vi "Filter From Source(Queue).vi"() -> ()   [LabVIEW 2017, in "CSM Global Log Filter Example.lvlib"]
uses:
  user.lib/_NEVSTOP/Communicable State Machine(CSM)/_Support/Typedef/_CSM_GlobalLog Filter Rules - v1.0.ctl
  user.lib/_NEVSTOP/Communicable State Machine(CSM)/_Support/Typedef/_CSM_GlobalLog_MSG_TYPE.ctl
  user.lib/_NEVSTOP/Communicable State Machine(CSM)/_Support/Typedef/_CSM_GlobalLog_STATE_TYPE.ctl
  user.lib/_NEVSTOP/Communicable State Machine(CSM)/Utility/_support/Periodic String Filter Level.ctl
  user.lib/_NEVSTOP/Communicable State Machine(CSM)/Utility/Periodic String Filter Setting.ctl
  user.lib/_NEVSTOP/Communicable State Machine(CSM)/_Support/GlobalEvent/GEvt-Set Source Filter Rules - v1.0.vi
  CSM Global Log Filter Example.lvlib
  user.lib/_NEVSTOP/Communicable State Machine(CSM)/Communicable State Machine.lvlib
  1. Create a reuse Module/1. Create a reuse Module.lvlib
  user.lib/_NEVSTOP/Communicable State Machine(CSM)/_Shared/CSM Shared.lvlib
panel:
  out "LogInQ":i32
  out "State History":string
  out "log handling Speed(#/s)":dbl
  out "LogInQ changing Speed(#/s)":dbl
  out "Level":T1
  in  "Stop":bool
  in  "Rules-v1":T2={"Global"={"CSM"=["Module2"], "LogType"=[], "State"=[], "StateType"=[]}, "CSM"={"LogType"=[{"CSM"="Module1", "LogType"=enum."State Change"}], "State"=[{"CSM"="Module3", "State"=""}], "StateType"=[]}}
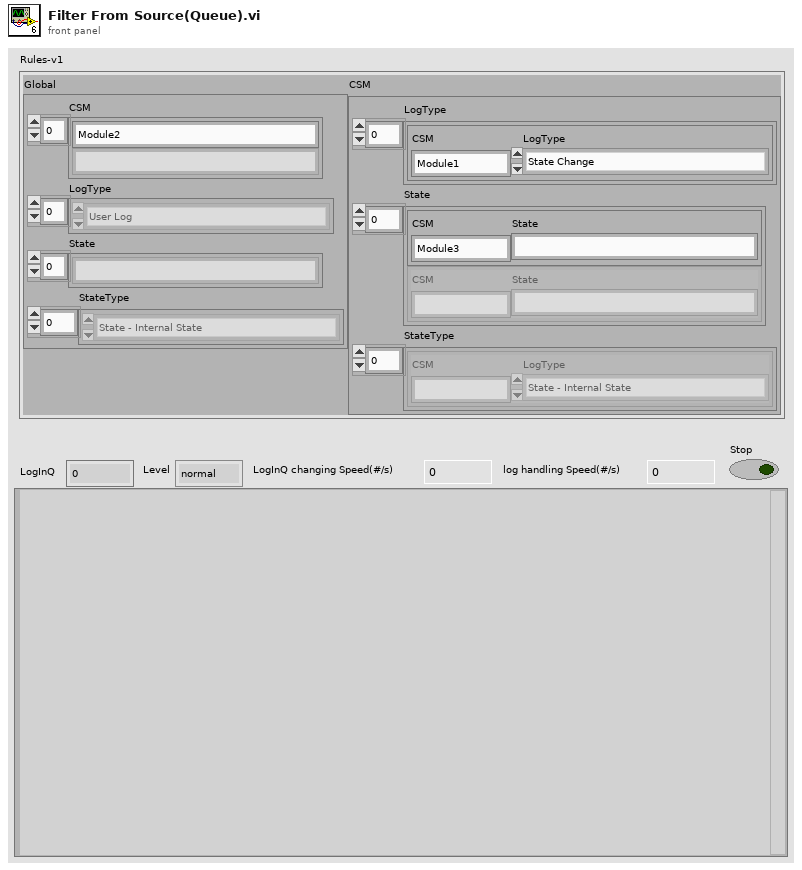
[diagram p1: front panel]
types:
  T1 = typedef "Communicable State Machine.lvlib/Periodic String Filter Level.ctl" = enum16{"normal", "L1", "L2", "L3", "L4"}
  T2 = typedef "Communicable State Machine.lvlib/_CSM_GlobalLog Filter Rules - v1.0.ctl" = cluster{"Global":cluster{"CSM":string[], "LogType":T3[], "State":string[], "StateType":T4[]}, "CSM":cluster{"LogType":cluster{"CSM":string, "LogType":T3}[], "State":cluster{"CSM":string, "State":string}[], "StateType":cluster{"CSM":string, "LogType":T4}[]}}
  T3 = typedef "Communicable State Machine.lvlib/_CSM_GlobalLog_MSG_TYPE.ctl" = enum16{"User Log", "State Change", "Status", "Interrupt", "Register", "Unregister", "Error Log", "Module Created", "Module Destroyed"}
  T4 = typedef "Communicable State Machine.lvlib/_CSM_GlobalLog_STATE_TYPE.ctl" = enum16{"State - Internal State", "State - External Message", "State - Response", "State - Complete"}
  T5 = typedef "Communicable State Machine.lvlib/Periodic String Filter Setting.ctl" = cluster{"threashold(#/s)":dbl, "Check Peroid(s)":dbl}
  T6 = typedef "Communicable State Machine.lvlib/_CSM_GlobalLog_MSG.ctl" = cluster{"Name (\"\" to Use UUID)":string, "Current State":string, "Arguments":string, "Source Message":T7, "Source Module":string, "Complete(T)/Start(F)":bool, "LogType":T3, "Time Stamp":timestamp}
  T7 = typedef "Communicable State Machine.lvlib/_CSM_Response Source Message.ctl" = cluster{"‘State":string, "’Arguments":string, "’Error":errorcluster}
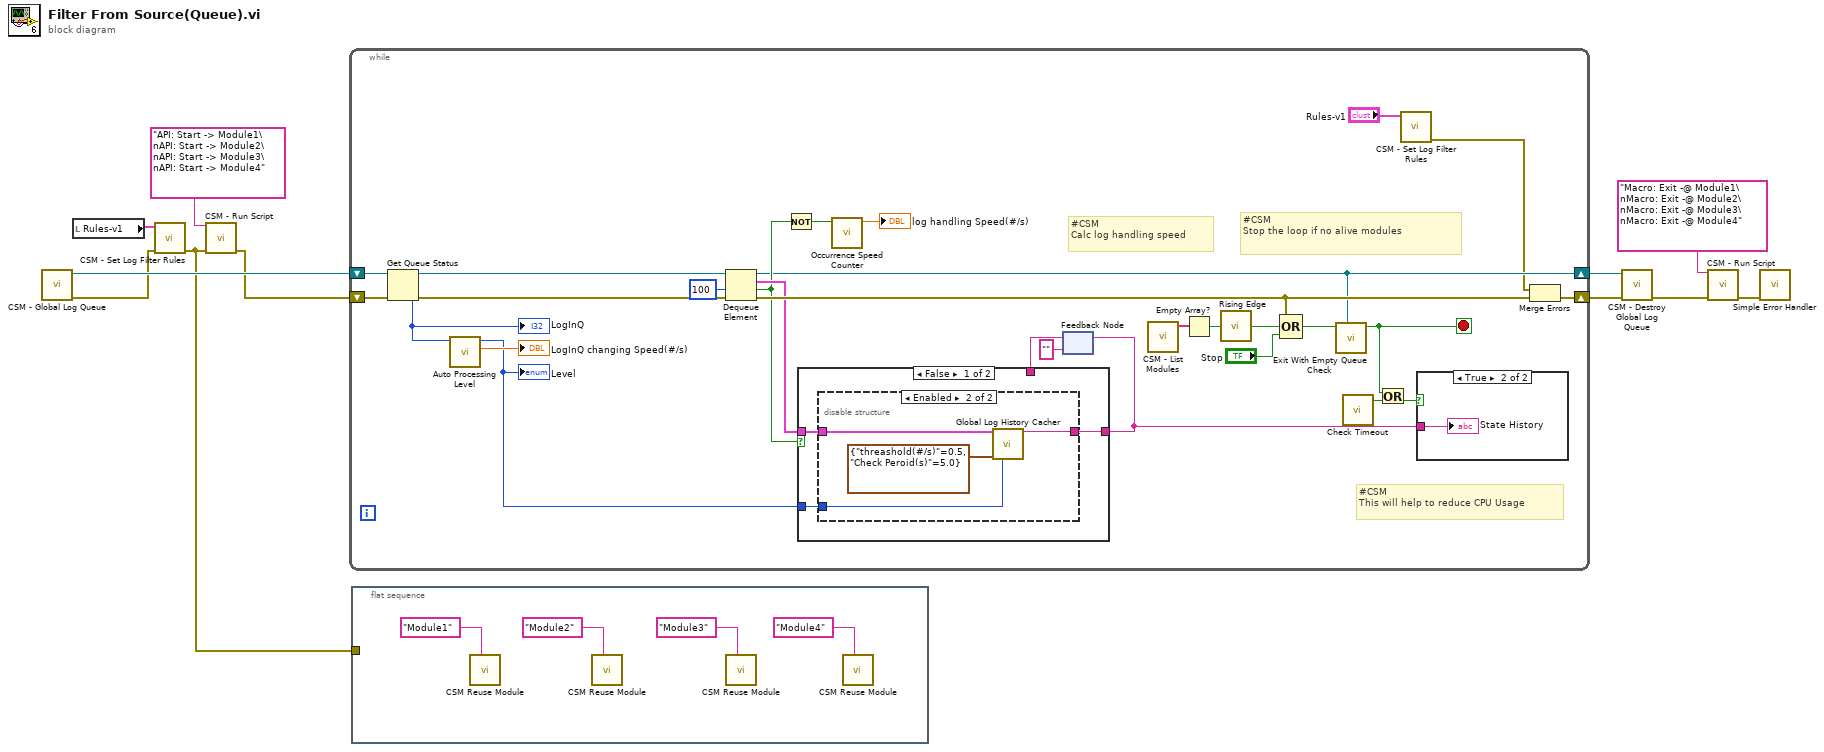
[diagram p0: block diagram]
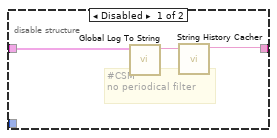
[diagram p2: hidden frame]
diagram:
  n1 = call "CSM - Global Log Queue.vi"() -> ("error out"=w6:errorcluster, "GlobalEvent Queue"=w7:refnum<queue>)  [unwired: 10 in]
  n2 = local read "Rules-v1"() -> (w11:T2)
  n3 = call-poly "CSM - Set Log Filter Rules.vi"("Error In"=w6, "Rules-v1"=w11) -> ("error out"=w4:errorcluster)  [unwired: 9 in]
  n4 = call "CSM - Run Script.vi"("CSM Scripts"="API: Start -> Module1\nAPI: Start -> Module2\nAPI: Start -> Module3\nAPI: Start -> Module4" ("single-line text"), "error in (no error)"=w4) -> ("error out"=w5:errorcluster)  [unwired: 11 in, 2 out]
  n5 = while {
    shift-right: [w14] -> w3
    shift-left: w5 -> [w35]
    shift-right: [w22] -> w8
    shift-left: w7 -> [w39]
    stop <- w12 stop-if-true
    # "#CSM\nCalc log handling speed"
    # "#CSM\nStop the loop if no alive modules"
    # "#CSM\nThis will help to reduce CPU Usage"
    n6 = Get Queue Status(queue=w39, error in (no error)=w35) -> (queue out=w37:refnum<queue>, error out=w36:errorcluster, # elements in queue=w18:i32)  [unwired: 1 in, 5 out]
    "LogInQ" <- w18
    n7 = call "Auto Processing Level.vi"("#Left In Q"=w18) -> ("LogInQ Changing Speed (#/s)"=→"LogInQ changing Speed(#/s)":dbl, "Level"=w17:T1)  [unwired: 8 in, 1 out]
    "Level" <- w17
    n8 = Dequeue Element(queue=w37, timeout in ms (-1)=100, error in (no error)=w36) -> (queue out=w22:refnum<queue>, element=w34:T6, timed out?=w24:bool, error out=w38:errorcluster)
    n9 = Not(x=w24) -> (.not. x?=w23:bool)
    n10 = call "Occurrence Speed Counter.vi"("Occured? (T)"=w23) -> ("Speed (#/s)"=→"log handling Speed(#/s)":dbl)  [unwired: 8 in, 2 out]
    n11 = feedback #1("" ("String Cache")) -> (w30:string)
    n12 = case shown="False" w24 {
      tunnel: w34 -> [w42 _]
      tunnel: [w41 w50] -> w31
      tunnel: w30 -> [_ w50]
      tunnel: w17 -> [w40 _]
      frame False {
        n13 = disable-structure shown="Enabled" {
          disable-tunnel: w42 -> [w45 w48]
          disable-tunnel: [w43 w49] -> w41
          disable-tunnel: w40 -> [_ w47]
          frame Disabled {
            # "#CSM \nno periodical filter"
            n14 = call "Global Log To String.vi"("Log"=w45) -> ("Log String"=w44:string)  [unwired: 9 in]
            n15 = call "String History Cacher.vi"("String"=w44) -> ("String Cache"=w43:string)  [unwired: 10 in]
          }
          frame Enabled {
            n16 = call "Global Log History Cacher.vi"("Cross CSM Data"=w48, "Settings"=T5 {"threashold(#/s)"=0.5, "Check Peroid(s)"=5.0}, "Level (Normal)"=w47) -> ("String Cache"=w49:string)  [unwired: 12 in]
          }
        }
      }
      frame True {
      }
    }
    n17 = feedback-in #1(w31) -> ()
    n18 = call "CSM - List Modules.vi"() -> ("Module Names"=w29:string[])  [unwired: 10 in, 1 out]
    n19 = Empty Array?(array=w29) -> (empty?=w28:bool)
    n20 = call "Rising Edge.vi"("Signal"=w28) -> ("Rising Edge"=w27:bool)
    n21 = Compound Arithmetic op=OR(w38, w27, "Stop") -> (w20:bool)
    n22 = call "Exit With Empty Queue Check.vi"("Queue"=w22, "Stop"=w20) -> ("Exit"=w12:bool)  [unwired: 8 in, 1 out]
    n23 = call "Check Timeout.vi"() -> ("Timeout"=w32:bool)  [unwired: 8 in]
    n24 = Or(x=w12, y=w32) -> (x .or. y?=w21:bool)
    n25 = call-poly "CSM - Set Log Filter Rules.vi"("Rules-v1"="Rules-v1") -> ("error out"=w13:errorcluster)  [unwired: 10 in]
    n26 = case shown="True" w21 {
      tunnel: w31 -> [_ w51]
      frame False {
      }
      frame True {
        "State History" <- w51
      }
    }
    n27 = Merge Errors(w13, w38) -> (w14:errorcluster)
  }
  n28 = flat-sequence {
    tunnel: w4 -> [_]
    frame #0 {
      n29 = call "CSM Reuse Module.vi"("Name (\"\" to Use UUID)"="Module1" ("Name(\"\" to use uuid)")) -> ()  [unwired: 11 in]
      n30 = call "CSM Reuse Module.vi"("Name (\"\" to Use UUID)"="Module2" ("Name(\"\" to use uuid)")) -> ()  [unwired: 11 in]
      n31 = call "CSM Reuse Module.vi"("Name (\"\" to Use UUID)"="Module3" ("Name(\"\" to use uuid)")) -> ()  [unwired: 11 in]
      n32 = call "CSM Reuse Module.vi"("Name (\"\" to Use UUID)"="Module4" ("Name(\"\" to use uuid)")) -> ()  [unwired: 11 in]
    }
  }
  n33 = call "CSM - Destroy Global Log Queue.vi"("Error In"=w3, "Global Log Queue"=w8) -> ("error out"=w2:errorcluster)  [unwired: 9 in]
  n34 = call "CSM - Run Script.vi"("CSM Scripts"="Macro: Exit -@ Module1\nMacro: Exit -@ Module2\nMacro: Exit -@ Module3\nMacro: Exit -@ Module4" ("single-line text"), "error in (no error)"=w2) -> ("error out"=w1:errorcluster)  [unwired: 11 in, 2 out]
  n35 = call <vilib>:"Simple Error Handler.vi"("error in (no error)"=w1) -> ()  [unwired: 4 in, 5 out]
